vi "Simple Teleop COde.vi"() -> ()   [LabVIEW 2017]
uses:
  <vilib>/Rock Robotics/WPI/Joystick/WPI_JoystickDeviceEnum.ctl
  <vilib>/Rock Robotics/SystemInterfaces/DIO/FPGA_DIOPWMChannel.ctl
  <vilib>/Rock Robotics/SystemInterfaces/DIO/FPGA_DIOChannel.ctl
  <vilib>/Rock Robotics/WPI/MotorControl/WPI_MotorControlOpen SPARK.vi
  <vilib>/Rock Robotics/WPI/Switch/WPI_SwitchOpenLimit.vi
  <vilib>/Rock Robotics/WPI/RobotDrive/WPI_RobotDriveOpen2MotorWithSPARK.vi
  <vilib>/Rock Robotics/WPI/RobotDrive/WPI_RobotDriveArcadeDrive_Standard(NoSaturation).vi
panel:
  in  "stop 2":bool
  out "Switch Pressed":bool
  out "Switch Pressed 2":bool
  in  "stop":bool
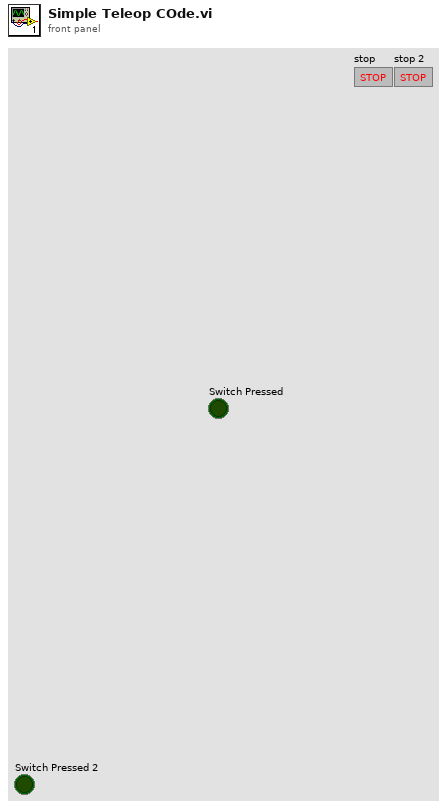
[diagram p1: front panel]
types:
  T1 = typedef "FPGA_DIOPWMChannel.ctl" = enum8{"PWM 0", "PWM 1", "PWM 2", "PWM 3", "PWM 4", "PWM 5", "PWM 6", "PWM 7", "PWM 8", "PWM 9", "PWM MXP 0", "PWM MXP 1", "PWM MXP 2", "PWM MXP 3", "PWM MXP 4", "PWM MXP 5", "PWM MXP 6", "PWM MXP 7", "PWM MXP 8", "PWM MXP 9", "Invalid"}
  T2 = typedef "FPGA_DIOChannel.ctl" = enum8{"DIO 0", "DIO 1", "DIO 2", "DIO 3", "DIO 4", "DIO 5", "DIO 6", "DIO 7", "DIO 8", "DIO 9", "DIO MXP 0", "DIO MXP 1", "DIO MXP 2", "DIO MXP 3", "DIO MXP 4", "DIO MXP 5", "DIO MXP 6", "DIO MXP 7", "DIO MXP 8", "DIO MXP 9", "DIO MXP 10", "DIO MXP 11", "DIO MXP 12", "DIO MXP 13", "DIO MXP 14", "DIO MXP 15", "SPI Port CS1", "SPI Port CS2", "SPI Port CS3", "SPI Port MISO", "SPI Port MOSI", "Invalid"}
  T3 = typedef "WPI_JoystickDeviceEnum.ctl" = enum16{"USB 0", "USB 1", "USB 2", "USB 3", "USB 4", "USB 5"}
  T4 = typedef "WPI_MotorControlDeviceRef.ctl" = cluster{"DeviceStatus":errorcluster, "Type":T5, "PWM":cluster{"PWM Channel":T1, "DeadBand":T6}, "CAN":cluster{"Device Number":u8, "SetOutput VI Ref":variant, "GetOutput VI Ref":variant, "Enable VI Ref":variant, "Disable VI Ref":variant, "Data":variant}, "Invert":bool, "DIO PWM":cluster{"PWM \"Enable\" Channel":T1, "DIOChannel":T2, "PWM Rate":dbl}}
  T5 = typedef "WPI_MotorControlType.ctl" = enum16{"PWM", "CAN", "DIO PWM"}
  T6 = typedef "WPI_PWMDeadband.ctl" = cluster{"Name":string, "maxPositivePwm":i32, "minPositivePwm":i32, "centerPwm":i32, "maxNegativePwm":i32, "minNegativePwm":i32, "angularRange":u16}
  T7 = typedef "WPI_SwitchDevRef.ctl" = cluster{"DevStatus":errorcluster, "DIO Channel":T2, "CntIndex":T8, "Normally Closed":bool}
  T8 = typedef "FPGA_CounterCtrSystemIndex.ctl" = enum8{"Ctr 0", "Ctr 1", "Ctr 2", "Ctr 3", "Ctr 4", "Ctr 5", "Ctr 6", "Ctr 7", "Invalid"}
  T9 = typedef "WPI_JoystickDevRef.ctl" = cluster{"Device":T3}
  T10 = typedef "WPI_RobotDriveDevRef.ctl" = cluster{"DevStatus":errorcluster, "Motors[]":T4[], "Square Inputs":bool, "Max Output":dbl}
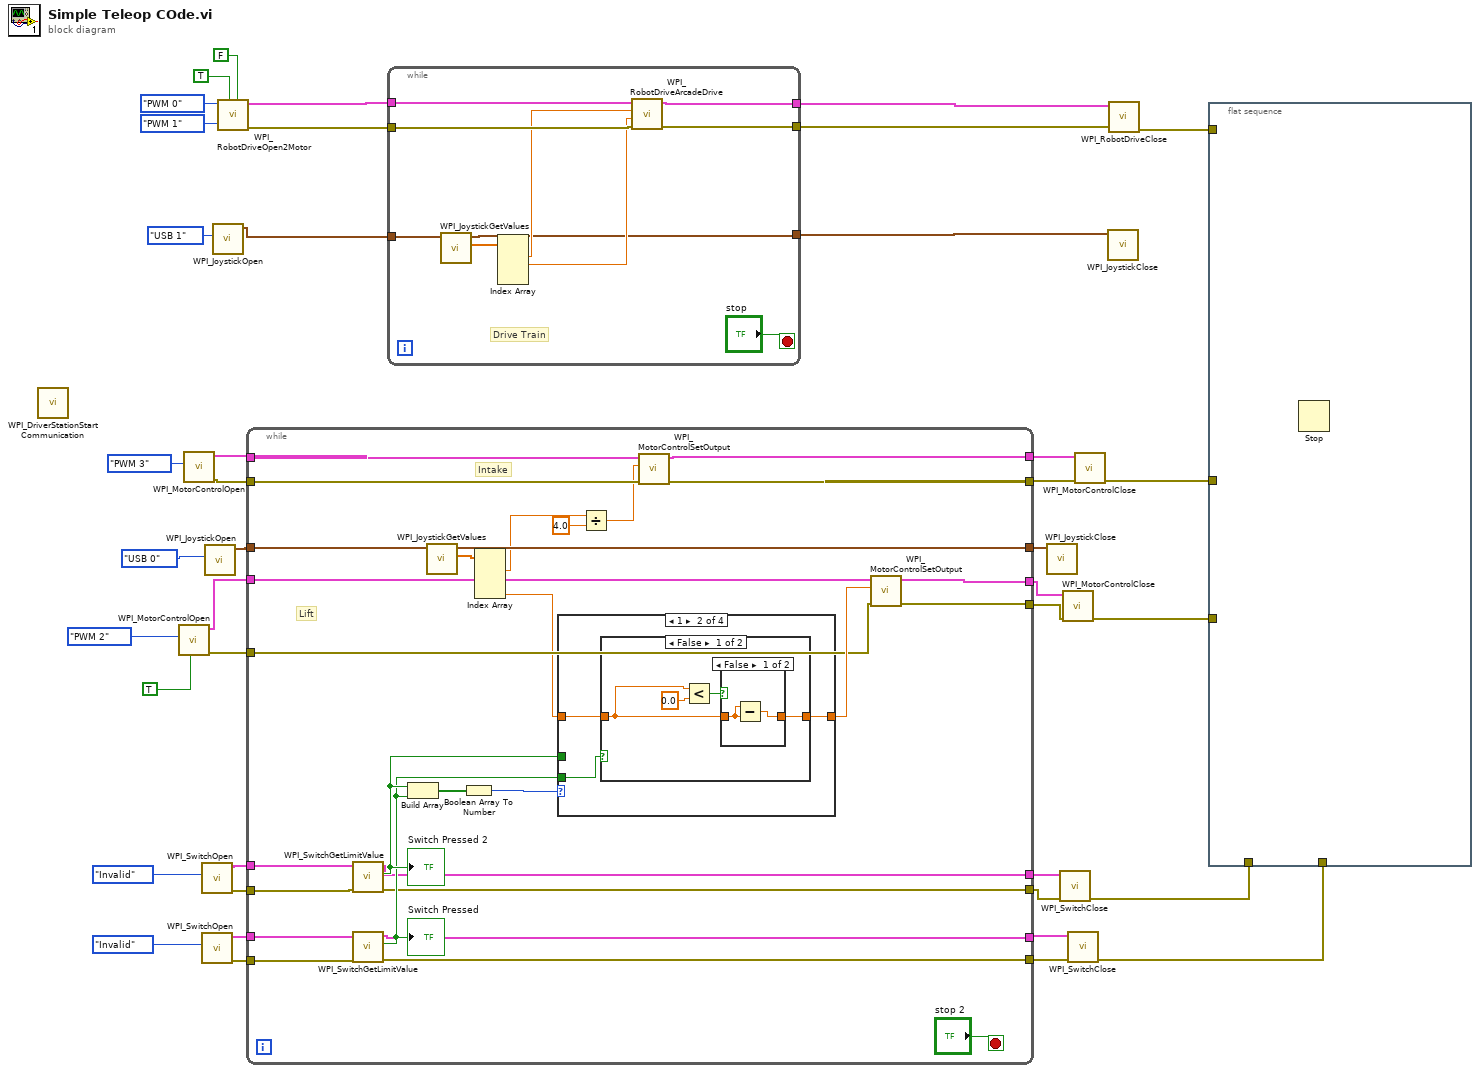
[diagram p0: block diagram]
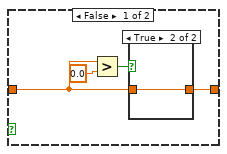
[diagram p6: hidden frame]
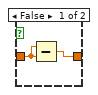
[diagram p7: hidden frame]
diagram:
  n1 = call <vilib>:"WPI_DriverStationStart Communication.vi"() -> ()  [unwired: 12 in]
  n2 = call-poly <vilib>:"WPI_MotorControlOpen.vi"("Invert"=TRUE, "PWM Channel"=FPGA_DIOPWMChannel."PWM 2" ("suck")) -> ("error out"=w14:errorcluster, "MotorControlDeviceRef"=w15:T4)  [unwired: 8 in]
  n3 = call-poly <vilib>:"WPI_MotorControlOpen.vi"("PWM Channel"=FPGA_DIOPWMChannel."PWM 3") -> ("error out"=w27:errorcluster, "MotorControlDeviceRef"=w30:T4)  [unwired: 9 in]
  n4 = call-poly <vilib>:"WPI_SwitchOpen.vi"("DIO Channel"=FPGA_DIOChannel."Invalid") -> ("error out"=w18:errorcluster, "SwitchDevRef"=w19:T7)  [unwired: 9 in]
  n5 = call-poly <vilib>:"WPI_SwitchOpen.vi"("DIO Channel"=FPGA_DIOChannel."Invalid") -> ("error out"=w16:errorcluster, "SwitchDevRef"=w17:T7)  [unwired: 9 in]
  n6 = call <vilib>:"WPI_JoystickOpen.vi"("JoystickDevice"=WPI_JoystickDeviceEnum."USB 0") -> ("JoystickDevRef"=w25:T9)  [unwired: 10 in]
  n7 = call <vilib>:"WPI_JoystickOpen.vi"("JoystickDevice"=WPI_JoystickDeviceEnum."USB 1") -> ("JoystickDevRef"=w40:T9)  [unwired: 10 in]
  n8 = call-poly <vilib>:"WPI_RobotDriveOpen2Motor.vi"("Right Motor Inverted"=FALSE, "Left Motor Inverted"=TRUE, "Right Motor"=FPGA_DIOPWMChannel."PWM 1", "Left Motor"=FPGA_DIOPWMChannel."PWM 0") -> ("error out"=w37:errorcluster, "RobotDriveDevRef"=w38:T10)  [unwired: 6 in]
  n9 = while {
    tunnel: w30 -> [w69]
    tunnel: [w68] -> w29
    tunnel: [w67] -> w28
    tunnel: w27 -> [w66]
    tunnel: w25 -> [w65]
    tunnel: [w63] -> w24
    tunnel: w19 -> [w57]
    tunnel: w18 -> [w56]
    tunnel: w17 -> [w55]
    tunnel: w16 -> [w54]
    tunnel: w15 -> [w53]
    tunnel: w14 -> [w52]
    tunnel: [w51] -> w8
    tunnel: [w50] -> w9
    tunnel: [w49] -> w13
    tunnel: [w48] -> w10
    tunnel: [w47] -> w11
    tunnel: [w46] -> w12
    stop <- "stop 2" stop-if-true
    # "Lift"
    # "Intake"
    n10 = call <vilib>:"WPI_SwitchGetLimitValue.vi"("error in (no error)"=w56, "SwitchDevRef"=w57) -> ("error out"=w48:errorcluster, "Switch Pressed"=w59:bool, "SwitchDevRef"=w49:T7)  [unwired: 7 in]
    "Switch Pressed 2" <- w59
    n11 = call <vilib>:"WPI_SwitchGetLimitValue.vi"("error in (no error)"=w54, "SwitchDevRef"=w55) -> ("error out"=w46:errorcluster, "Switch Pressed"=w58:bool, "SwitchDevRef"=w47:T7)  [unwired: 7 in]
    "Switch Pressed" <- w58
    n12 = Build Array(w59, w58) -> (w62:bool[])
    n13 = call <vilib>:"WPI_JoystickGetValues.vi"("JoystickDevRef"=w65) -> ("Axes"=w64:dbl[], "JoystickDevRef"=w63:T9)  [unwired: 6 in, 3 out]
    n14 = Boolean Array To Number(Boolean array=w62) -> (number=w61:u32)
    n15 = Index Array(array=w64) -> (element #1=w42:dbl, element #4=w41:dbl)  [unwired: 4 in, 2 out]
    n16 = case shown="1" w61 {
      tunnel: [w70 w73 w84 w93] -> w60
      tunnel: w58 -> [_ w72 _ _]
      tunnel: w59 -> [_ _ w83 _]
      tunnel: w41 -> [w70 w71 w82 w93]
      frame 0, Default {
      }
      frame 1 {
        n17 = case shown="False" w72 {
          tunnel: [w75 w81] -> w73
          tunnel: w71 -> [w74 w81]
          frame False {
            n18 = Less?(x=w74, y=0.0) -> (x < y?=w76:bool)
            n19 = case shown="False" w76 {
              tunnel: [w79 w80] -> w75
              tunnel: w74 -> [w78 w80]
              frame False {
                n20 = Subtract(x=w78, y=w78) -> (x-y=w79:dbl)
              }
              frame True {
              }
            }
          }
          frame True {
          }
        }
      }
      frame 2 {
        n21 = case shown="True" w83 {
          tunnel: [w86 w92] -> w84
          tunnel: w82 -> [w85 w92]
          frame False {
            n22 = Greater?(x=w85, y=0.0) -> (0:w87:bool)
            n23 = case shown="True" w87 {
              tunnel: [w90 w91] -> w86
              tunnel: w85 -> [w89 w91]
              frame False {
                n24 = Subtract(x=w89, y=w89) -> (x-y=w90:dbl)
              }
              frame True {
              }
            }
          }
          frame True {
          }
        }
      }
      frame 3 {
      }
    }
    n25 = Divide(x=w42, y=4.0) -> (x/y=w44:dbl)
    n26 = call <vilib>:"WPI_MotorControlSetOutput.vi"("error in (no error)"=w66, "Output"=w44, "MotorControlDevRef"=w69) -> ("error out"=w67:errorcluster, "MotorControlDevRef"=w68:T4)  [unwired: 6 in, 1 out]
    n27 = call <vilib>:"WPI_MotorControlSetOutput.vi"("error in (no error)"=w52, "Output"=w60, "MotorControlDevRef"=w53) -> ("error out"=w51:errorcluster, "MotorControlDevRef"=w50:T4)  [unwired: 6 in, 1 out]
  }
  n28 = while {
    tunnel: w40 -> [w102]
    tunnel: w38 -> [w101]
    tunnel: w37 -> [w100]
    tunnel: [w96] -> w34
    tunnel: [w95] -> w33
    tunnel: [w94] -> w32
    stop <- "stop" stop-if-true
    # "Drive Train"
    n29 = call <vilib>:"WPI_JoystickGetValues.vi"("JoystickDevRef"=w102) -> ("Axes"=w99:dbl[], "JoystickDevRef"=w94:T9)  [unwired: 6 in, 3 out]
    n30 = Index Array(array=w99) -> (element #1=w98:dbl, element #2=w97:dbl)  [unwired: 4 in, 2 out]
    n31 = call-poly <vilib>:"WPI_RobotDriveArcadeDrive.vi"("error in (no error)"=w100, "Y axis value"=w97, "X axis value"=w98, "RobotDriveDevRef"=w101) -> ("error out"=w95:errorcluster, "RobotDriveDevRef"=w96:T10)  [unwired: 5 in, 1 out]
  }
  n32 = call <vilib>:"WPI_JoystickClose.vi"("JoystickDevRef"=w24) -> ()  [unwired: 11 in]
  n33 = call <vilib>:"WPI_SwitchClose.vi"("error in (no error)"=w10, "SwitchDevRef"=w13) -> ("error out"=w5:errorcluster)  [unwired: 9 in]
  n34 = call <vilib>:"WPI_MotorControlClose.vi"("error in"=w8, "MotorControlDevRef"=w9) -> ("error out"=w1:errorcluster)  [unwired: 9 in]
  n35 = call <vilib>:"WPI_SwitchClose.vi"("error in (no error)"=w12, "SwitchDevRef"=w11) -> ("error out"=w4:errorcluster)  [unwired: 9 in]
  n36 = call <vilib>:"WPI_MotorControlClose.vi"("error in"=w28, "MotorControlDevRef"=w29) -> ("error out"=w2:errorcluster)  [unwired: 9 in]
  n37 = call <vilib>:"WPI_JoystickClose.vi"("JoystickDevRef"=w32) -> ()  [unwired: 11 in]
  n38 = call <vilib>:"WPI_RobotDriveClose.vi"("error in (no error)"=w33, "RobotDriveDevRef"=w34) -> ("error out"=w3:errorcluster)  [unwired: 9 in]
  n39 = flat-sequence {
    tunnel: w5 -> [_]
    tunnel: w4 -> [_]
    tunnel: w3 -> [_]
    tunnel: w2 -> [_]
    tunnel: w1 -> [_]
    frame #0 {
      n40 = Stop() -> ()  [unwired: 1 in]
    }
  }
